vi "2x2QAMAlamouti with BER.vi"() -> ()   [LabVIEW 2011]
uses:
  usrpHardwareSettings.ctl
  <instrlib>/niUSRP/niUSRP Timestamp.ctl
  ModulationParameters.ctl
  <vilib>/addons/Modulation/Digital/General/MT Generate Bits (Galois, PN Order).vi
  <vilib>/addons/Modulation/Digital/General/MT Map Bits to PSK Symbols.vi
  <vilib>/addons/Modulation/Digital/General/MT Map PSK Symbols to Bits.vi
  <vilib>/addons/Modulation/Digital/Demodulation/MT Calculate BER After Trigger (PN Sequence).vi
  <vilib>/addons/Modulation/niDMT.lvlib
panel:
  in  "Tab Control 2":T1(tab)
  in  "Link Parameters":T2={"Symbol Rate"=1000000.0, "Symbols per Packet"=2000, "Tx Oversample Factor"=12, "Rx Oversample Factor"=12, "Modulation Scheme"=enum."4-QAM", "filter length (symbols)"=4, "filter parameter"=0.5, "Training Sequence"=[0.7071067811865475+0.7071067811865475i, 0.7071067811865475+0.7071067811865475i, 0.7071067811865475+0.7071067811865475i, -0.7071067811865475-0.7071067811865475i, -0.7071067811865475-0.7071067811865475i, -0.7071067811865475-0.7071067811865475i, 0.7071067811865475+0.7071067811865475i, -0.7071067811865475-0.7071067811865475i, -0.7071067811865475-0.7071067811865475i, 0.7071067811865475+0.7071067811865475i, -0.7071067811865475-0.7071067811865475i, 0.7071067811865475+0.7071067811865475i, 0.7071067811865475+0.7071067811865475i, 0.7071067811865475+0.7071067811865475i, -0.7071067811865475-0.7071067811865475i, -0.7071067811865475-0.7071067811865475i, -0.7071067811865475-0.7071067811865475i, 0.7071067811865475+0.7071067811865475i, -0.7071067811865475-0.7071067811865475i, -0.7071067811865475-0.7071067811865475i, 0.7071067811865475+0.7071067811865475i, -0.7071067811865475-0.7071067811865475i, 0.7071067811865475+0.7071067811865475i, 0.7071067811865475+0.7071067811865475i, 0.7071067811865475+0.7071067811865475i, -0.7071067811865475-0.7071067811865475i, -0.7071067811865475-0.7071067811865475i, -0.7071067811865475-0.7071067811865475i, 0.7071067811865475+0.7071067811865475i, -0.7071067811865475-0.7071067811865475i, -0.7071067811865475-0.7071067811865475i, 0.7071067811865475+0.7071067811865475i, -0.7071067811865475-0.7071067811865475i, 0.7071067811865475+0.7071067811865475i, 0.7071067811865475+0.7071067811865475i, 0.7071067811865475+0.7071067811865475i, -0.7071067811865475-0.7071067811865475i, -0.7071067811865475-0.7071067811865475i, -0.7071067811865475-0.7071067811865475i, 0.7071067811865475+0.7071067811865475i, -0.7071067811865475-0.7071067811865475i, -0.7071067811865475-0.7071067811865475i, 0.7071067811865475+0.7071067811865475i, -0.7071067811865475-0.7071067811865475i], "Channel Length Estimate"=2, "Frequency Offset\nCorrection?"=FALSE} {"Symbol Rate" format="%#_6p"; "Training Sequence" format="%#_3p"; "filter parameter" format="%.2f"}
  in  "Rx Settings":T3={"USRP IP Address"="192.168.10.14;192.168.10.15", "IQ Sampling\nRate [S/sec]"=12000000.0, "Carrier Frequency [Hz]"=438200000.0, "Start Trigger Time"={"whole seconds"=4, "fractional seconds"=0.0}, "Per Device"=[{"active antenna"="RX1", "gain"=10.0, "Ref Frequency Source"="RefIn", "Timebase Clock Source"="PpsIn"}, {"active antenna"="RX1", "gain"=10.0, "Ref Frequency Source"="Mimo", "Timebase Clock Source"="Mimo"}]} {"Per Device"."gain" format="%#_6f"; "Carrier Frequency [Hz]" min=50000000.0 max=6000000000.0 step=1000.0 format="%#.15p"; "IQ Sampling\nRate [S/sec]" format="%#_6p"}
  in  "Tx Settings":T3={"USRP IP Address"="192.168.10.2;192.168.10.3", "IQ Sampling\nRate [S/sec]"=12000000.0, "Carrier Frequency [Hz]"=438200000.0, "Start Trigger Time"={"whole seconds"=4, "fractional seconds"=0.0002}, "Per Device"=[{"active antenna"="TX1", "gain"=10.0, "Ref Frequency Source"="RefIn", "Timebase Clock Source"="PpsIn"}, {"active antenna"="TX1", "gain"=10.0, "Ref Frequency Source"="Mimo", "Timebase Clock Source"="Mimo"}]} {"Per Device"."gain" format="%#_6f"; "Carrier Frequency [Hz]" min=50000000.0 max=6000000000.0 step=1000.0 format="%#.15p"; "IQ Sampling\nRate [S/sec]" format="%#_6p"}
  out "error out":errorcluster
  out "Combined Rx":T5(graph)
  out "Rx Channel 2":T5(graph)
  out "Rx Channel 1":T5(graph)
  out "Rx Signal (Time Domain)":dbl[][](graph)
  out "BER":dbl format="%.4f"
  out "trigger found?":bool=TRUE
  out "output bit stream":i8[](array[numeric])
  out "input bit stream":i8[](array[numeric])
  # "2x2 Alamouti Coding"
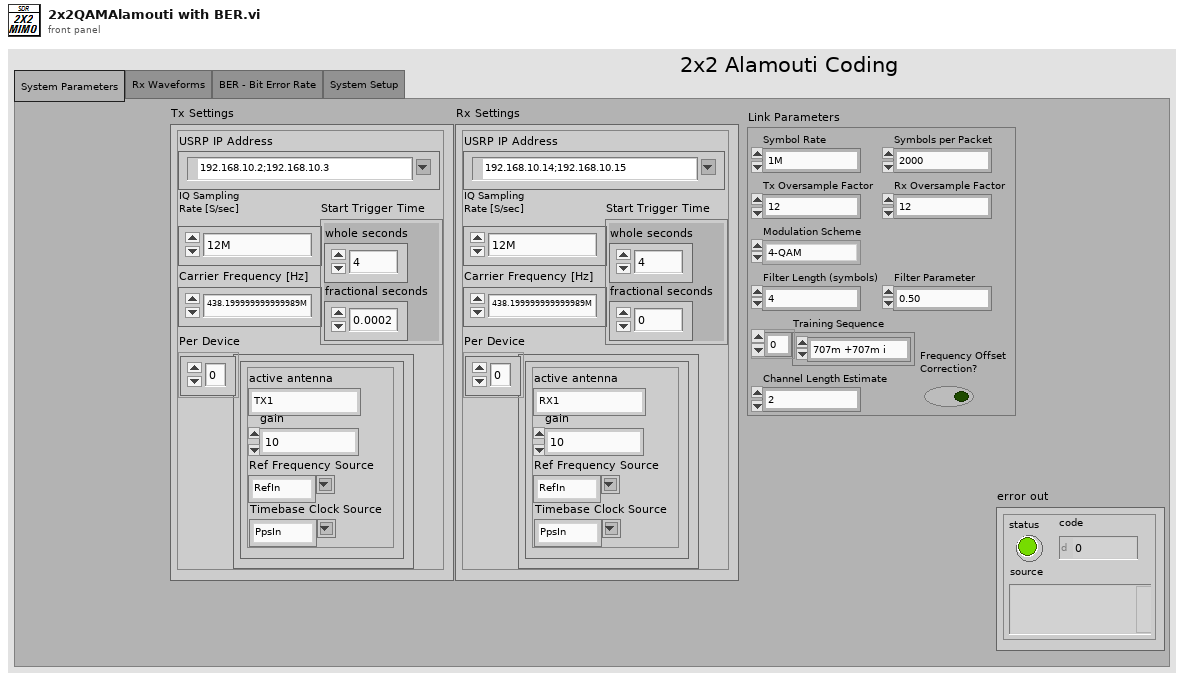
[diagram p1: front panel]
types:
  T1 = enum32{"System Parameters", "Rx Waveforms", "BER - Bit Error Rate", "System Setup"}
  T2 = typedef "ModulationParameters.ctl" = cluster{"Symbol Rate":dbl, "Symbols per Packet":i32, "Tx Oversample Factor":i32, "Rx Oversample Factor":i32, "Modulation Scheme":enum16{"4-QAM", "16-QAM", "64-QAM"}, "filter length (symbols)":i32, "filter parameter":dbl, "Training Sequence":cdb[], "Channel Length Estimate":i32, "Frequency Offset\nCorrection?":bool}
  T3 = typedef "usrpHardwareSettings.ctl" = cluster{"USRP IP Address":refnum<k15>, "IQ Sampling\nRate [S/sec]":dbl, "Carrier Frequency [Hz]":dbl, "Start Trigger Time":T4, "Per Device":cluster{"active antenna":string, "gain":dbl, "Ref Frequency Source":string, "Timebase Clock Source":string}[]}
  T4 = typedef "niUSRP Timestamp.ctl" = cluster{"whole seconds":u64, "fractional seconds":dbl}
  T5 = cluster{"constellation":dbl[], "oversampled data":dbl[]}[]
  T6 = typedef "CalculatedParameters.ctl" = cluster{"Symbol Map":cdb[], "bits/symbol":i32, "pulse shaping filter coefficients":dbl[], "matched filter coefficients":dbl[]}
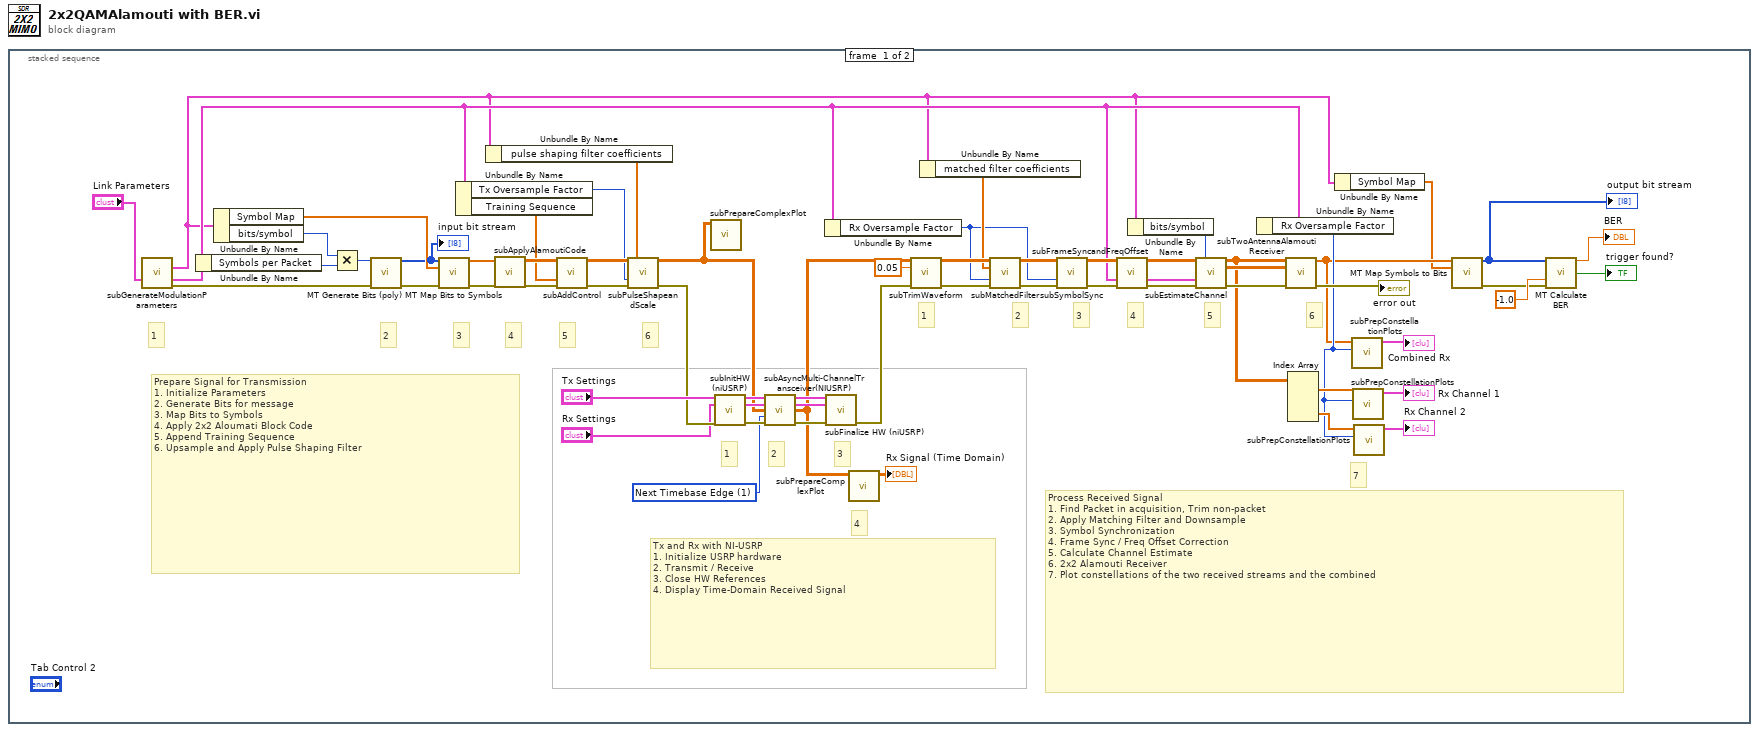
[diagram p0: block diagram]
diagram:
  n1 = stacked-sequence {
    frame #0 {
      w12 = 1 items=["Now", "Next Timebase Edge"] ("apply timestamp")
      # "Process Received Signal\n1. Find Packet in acquisition, Trim non-packet\n2. Apply Matching Filter and Downsample\n3. Symbol Synchronization\n4. Frame Sync / Freq Offset Correction\n5. Calculate Channel Estimate\n6. 2x2 Alamouti Receiver\n7. Plot constellations of the two received streams and the combined"
      # "7"
      # "6"
      # "5"
      # "4"
      # "3"
      # "2"
      # "1"
      # "4"
      # "3"
      # "2"
      # "1"
      # "6"
      # "5"
      # "4"
      # "3"
      # "2"
      # "1"
      # "Prepare Signal for Transmission\n1. Initialize Parameters\n2. Generate Bits for message\n3. Map Bits to Symbols\n4. Apply 2x2 Aloumati Block Code\n5. Append Training Sequence\n6. Upsample and Apply Pulse Shaping Filter"
      # "Tx and Rx with NI-USRP\n1. Initialize USRP hardware\n2. Transmit / Receive\n3. Close HW References\n4. Display Time-Domain Received Signal"
      n2 = call "subGenerateModulationParameters.vi"("System Parameters"="Link Parameters") -> ("Calculated Parameters"=w5:T6, "System Parameters (out)"=w14:T2, "error out"=w23:errorcluster)  [unwired: 12 in]
      n3 = Unbundle By Name(w14) -> ("Symbols per Packet"=w44:i32)
      n4 = Unbundle By Name(w5) -> ("Symbol Map"=w45:cdb[], "bits/symbol"=w43:i32)
      n5 = Multiply(x=w43, y=w44) -> (x*y=w46:i32)
      n6 = call-poly <vilib>:"MT Generate Bits (poly).vi"("total bits (128)"=w46, "error in (no error)"=w23) -> ("output bit stream"=w1:i8[], "error out"=w52:errorcluster)  [unwired: 4 in, 8 out]
      "input bit stream" <- w1
      n7 = call-poly <vilib>:"MT Map Bits to Symbols.vi"("input bit stream"=w1, "symbol map"=w45, "error in (no error)"=w52) -> ("symbols"=w47:cdb[], "error out"=w54:errorcluster)  [unwired: 11 in]
      n8 = Unbundle By Name(w14) -> ("Tx Oversample Factor"=w39:i32, "Training Sequence"=w40:cdb[])
      n9 = Unbundle By Name(w5) -> ("pulse shaping filter coefficients"=w38:dbl[])
      n10 = call "subApplyAlamoutiCode.vi"("Modulated Stream"=w47) -> ("Baseband Streams"=w55:cdb[][])  [unwired: 10 in]
      n11 = call "subAddControl.vi"("Input Symbol Stream"=w55, "Training Sequence"=w40, "error in (no error)"=w54) -> ("Output Transmit \nPackets"=w42:cdb[][], "error out"=w41:errorcluster)  [unwired: 11 in]
      n12 = call "subPulseShapeandScale.vi"("Symbol Stream"=w42, "pulse shaping filter coefficients"=w38, "samples per symbol (16)"=w39, "error in (no error)"=w41) -> ("Transmit Packets"=w11:cdb[][], "error out"=w31:errorcluster)  [unwired: 10 in]
      n13 = call "subPrepareComplexPlot.vi"("Array in"=w11) -> ()  [unwired: 10 in, 1 out]
      n14 = call "subInitHW (niUSRP).vi"("Tx Settings"="Tx Settings", "Rx Settings"="Rx Settings", "error in (no error)"=w31) -> ("Tx Settings (out)"=w61:T3, "Rx Settings (out)"=w60:T3, "error out"=w59:errorcluster)  [unwired: 10 in]
      n15 = call "subAsyncMulti-ChannelTransceiver(NIUSRP).vi"("Tx Settings"=w61, "Rx Settings"=w60, "Tx Waveforms"=w11, "apply timestamp"=w12, "error in (no error)"=w59) -> ("Tx Settings (out)"=w57:T3, "Rx Settings (out)"=w58:T3, "Rx Waveforms"=w48:cdb[][], "error out"=w51:errorcluster)  [unwired: 7 in]
      n16 = Unbundle By Name(w14) -> ("Rx Oversample Factor"=w15:i32)
      n17 = call "subFinalize HW (niUSRP).vi"("Tx Settings"=w57, "Rx Settings"=w58, "error in (no error)"=w51) -> ("error out"=w50:errorcluster)  [unwired: 12 in]
      n18 = call "subPrepareComplexPlot.vi"("Array in"=w48) -> ("Array out"=→"Rx Signal (Time Domain)":dbl[][])  [unwired: 10 in]
      n19 = call "subTrimWaveform.vi"("input waveform"=w48, "magnitude threshold (of peak)"=0.05, "error in (no error)"=w50) -> ("output waveform"=w28:cdb[][], "error out"=w26:errorcluster)  [unwired: 11 in]
      n20 = Unbundle By Name(w5) -> ("matched filter coefficients"=w27:dbl[])
      n21 = call "subMatchedFilter.vi"("Symbol Stream"=w28, "pulse shaping filter coefficients"=w27, "samples per symbol (16)"=w15, "error in (no error)"=w26) -> ("Transmit Packets"=w24:cdb[][], "error out"=w25:errorcluster)  [unwired: 10 in]
      n22 = call "subSymbolSync.vi"("Data stream"=w24, "Rx Oversample Factor"=w15, "error in (no error)"=w25) -> ("Data stream (out)"=w29:cdb[][], "error out"=w37:errorcluster)  [unwired: 11 in]
      n23 = call "subFrameSyncandFreqOffset.vi"("Data stream"=w29, "System Parameters"=w14, "error in (no error)"=w37) -> ("Data stream (out)"=w34:cdb[][], "System Parameters (out)"=w36:T2, "error out"=w35:errorcluster)  [unwired: 8 in, 2 out]
      n24 = Unbundle By Name(w5) -> ("bits/symbol"=w13:i32)
      n25 = call "subEstimateChannel.vi"("Data Stream In"=w34, "bits/symbol"=w13, "System Parameters"=w36, "error in (no error)"=w35) -> ("Symbols Out"=w16:cdb[][], "h[n]"=w32:cdb[][][], "error out"=w33:errorcluster)  [unwired: 9 in]
      n26 = Unbundle By Name(w14) -> ("Rx Oversample Factor"=w18:i32)
      n27 = call "subTwoAntennaAlamoutiReceiver.vi"("symbols in"=w16, "channel estimate"=w32, "error in (no error)"=w33) -> ("symbols out"=w9:cdb[], "error out"=→"error out":errorcluster)  [unwired: 11 in]
      n28 = Index Array(array=w16) -> (element #1=w22:cdb[], element #2=w19:cdb[])  [unwired: 4 in]
      n29 = Unbundle By Name(w5) -> ("Symbol Map"=w4:cdb[])
      n30 = call "subPrepConstellationPlots.vi"("Oversample Factor"=w18, "Y"=w9) -> ("constellation graph"=→"Combined Rx":T5)  [unwired: 9 in]
      n31 = call "subPrepConstellationPlots.vi"("Oversample Factor"=w18, "Y"=w22) -> ("constellation graph"=→"Rx Channel 1":T5)  [unwired: 9 in]
      n32 = call "subPrepConstellationPlots.vi"("Oversample Factor"=w18, "Y"=w19) -> ("constellation graph"=→"Rx Channel 2":T5)  [unwired: 9 in]
      n33 = call-poly <vilib>:"MT Map Symbols to Bits.vi"("symbols"=w9, "symbol map"=w4) -> ("output bit stream"=w7:i8[], "error out"=w3:errorcluster)  [unwired: 5 in, 7 out]
      "output bit stream" <- w7
      n34 = call-poly <vilib>:"MT Calculate BER.vi"("input bit stream"=w7, "confidence (0.95)"=-1.0, "error in (no error)"=w3) -> ("BER"=→"BER":dbl, "trigger found?"=→"trigger found?":bool)  [unwired: 8 in, 3 out]
    }
    frame #1 {
    }
  }
